vi "Get Monotonically Increasing State Name.vi"(8 "error in (no error)":errorcluster, 10 "State Names":string[](array[string]), 11 "Desired State Name":string) -> (0 "error out":errorcluster, 3 "New State Name":string)   [LabVIEW 2019, in "Routing and Faulting System Explorer.lvlib"]
uses:
  Routing and Faulting System Explorer.lvlib
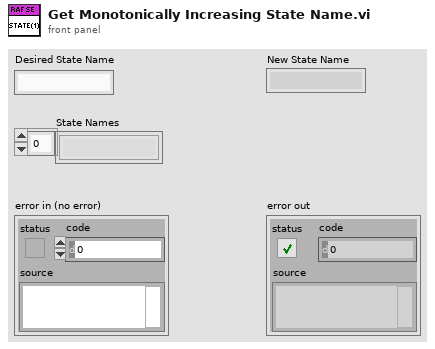
[diagram p1: front panel]
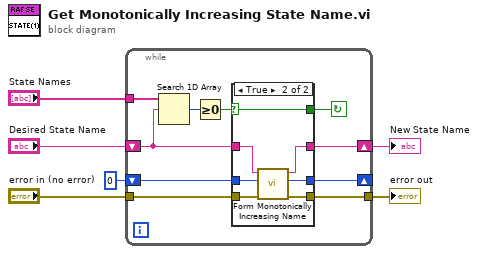
[diagram p0: block diagram]
diagram:
  n1 = while {
    tunnel: "error in (no error)" -> [w12]
    shift-right: [w15] -> w3
    shift-left: "Desired State Name" -> [w7]
    shift-right: [w16] -> _
    shift-left: 0 ("y") -> [w11]
    tunnel: [w14] -> w2
    tunnel: "State Names" -> [w10]
    stop <- w13 continue-if-true
    n2 = Search 1D Array(1D array=w10, element=w7) -> (index of element=w9:i32)  [unwired: 1 in]
    n3 = Greater Or Equal To 0?(x=w9) -> (x >= 0?=w8:bool)
    n4 = case shown="True" w8 {
      selector: w8 -> [w17 w21]
      tunnel: w7 -> [w19 w26]
      tunnel: w12 -> [w18 w24]
      tunnel: w11 -> [w20 w27]
      tunnel: [w20 w22] -> w16
      tunnel: [w19 w25] -> w15
      tunnel: [w18 w23] -> w14
      tunnel: [w17 w21] -> w13
      frame False {
      }
      frame True {
        n5 = call "Form Monotonically Increasing Name.vi"("error in (no error)"=w24, "index"=w27, "Desired Name"=w26) -> ("error out"=w23:errorcluster, "next index"=w22:i32, "Next Candidate Name"=w25:string)  [unwired: 6 in]
      }
    }
  }
  "New State Name" <- w3
  "error out" <- w2
